vi "AO_6738_Load_Wfm.vi"(8 "error in (no error)":errorcluster, 9 "SOFTWARE Inputs":T2={"Application Directory"=path "D:/S.O.F.T.S/LABVIEW/PIL", "Software Version"="1.0.0", "Data Path"=path "D:/PIRENEA/DATA", "XML Path"=path "D:/PIRENEA/DATA", "XML File Filter"="*.xml", "XML Saved Path"=path "D:/PIRENEA/DATA/SAVED", "Excit Scripts Path"=path "D:/PIRENEA/TECHNICAL/EXCIT_SCRIPTS", "Excit Scripts File Filter"="*.txt", "Excit Waveforms Path"=path "D:/PIRENEA/TECHNICAL/EXCIT_WFMS", "Excit Waveforms File Filter"="*.bin", "Timing Scripts Path"=path "D:/PIRENEA/TECHNICAL/TIMING_SCRIPTS", "Timing Scripts File Filter"="*.txt", "Timing Waveforms Path"=path "D:/PIRENEA/TECHNICAL/TIMING_WFMS", "Timing Waveforms File Filter"="*.bin", "Trapping Waveforms Path"=path "D:/PIRENEA/TECHNICAL/TRAPPING_WFMS", "Trapping Waveforms File Filter"="*.bin"}, 10 "RF_TRAPPING Inputs":T1={"Init Values"=[0.0, 1.0, 1.0, 0.0], "Opening Values"=[0.0, -4.0, 1.0, 0.0], "Trapping Values"=[0.0, 1.0, 1.0, 0.0], "Emptying Values"=[0.0, 1.0, -7.0, 0.0], "RF Trap ON"=FALSE, "RF Accums"=1, "Number of Voltages"=4} {"RF Accums" min=1 max=100; "Trapping Values" min=-10.0 max=10.0; "Init Values" min=-10.0 max=10.0; "Emptying Values" min=-10.0 max=10.0; "Opening Values" min=-10.0 max=10.0}, 11 "Instrument handle in":refnum<k21> caption="tâche/voies en entrée") -> (0 "error out":errorcluster, 1 "number of samples written per channel":u32 caption="nombre d'échantillons écrits par voie", 2 "number of samples":i32, 3 "Instrument handle out":refnum<k21>)   [LabVIEW 2024]
doc: "This VI demonstrates how to load dynamic waveforms into the board.\n\n1. The waveform binary files are read one by one from the waveform folder.\n2. The data are converted to U32 format and loaded into the on-board memory.\n\nThis VI returns the max memory size of the board, the memory used after loading, and a list of the waveforms loaded. No check of memory overflow is done."
uses:
  controls/SOFTWARE_Inputs.ctl
  controls/RF_TRAPPING_Inputs.ctl
  <vilib>/DAQmx/write.llb/DAQmx Write (Analog 2D DBL NChan NSamp).vi
  <vilib>/DAQmx/miscellaneous.llb/DAQmx Fill In Error Info.vi
  <resource>/objmgr/daqmx.rc
panel:
  # "RF_V1"
  # "RF_V2"
  # "RF_V3"
  # "RF_V4"
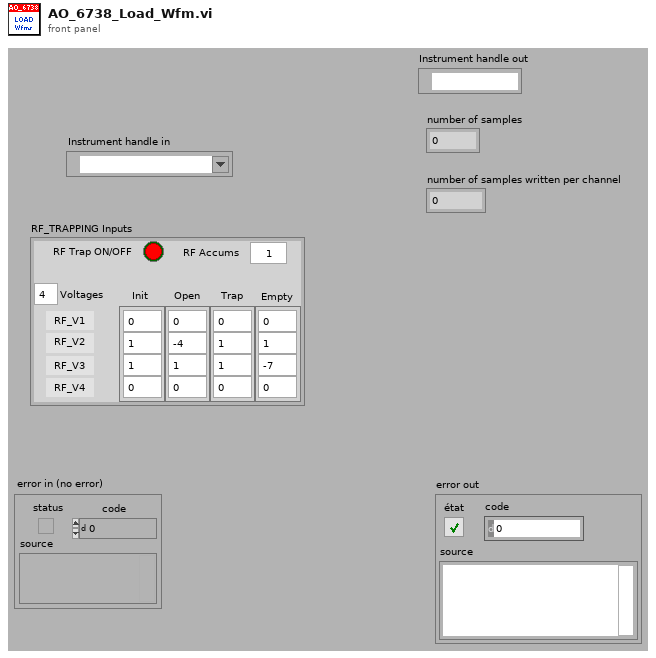
[diagram p1: front panel]
types:
  T1 = typedef "RF_TRAPPING_Inputs.ctl" = cluster{"Init Values":dbl[], "Opening Values":dbl[], "Trapping Values":dbl[], "Emptying Values":dbl[], "RF Trap ON":bool, "RF Accums":i32, "Number of Voltages":i32}
  T2 = typedef "SOFTWARE_Inputs.ctl" = cluster{"Application Directory":path, "Software Version":string, "Data Path":path, "XML Path":path, "XML File Filter":string, "XML Saved Path":path, "Excit Scripts Path":path, "Excit Scripts File Filter":string, "Excit Waveforms Path":path, "Excit Waveforms File Filter":string, "Timing Scripts Path":path, "Timing Scripts File Filter":string, "Timing Waveforms Path":path, "Timing Waveforms File Filter":string, "Trapping Waveforms Path":path, "Trapping Waveforms File Filter":string}
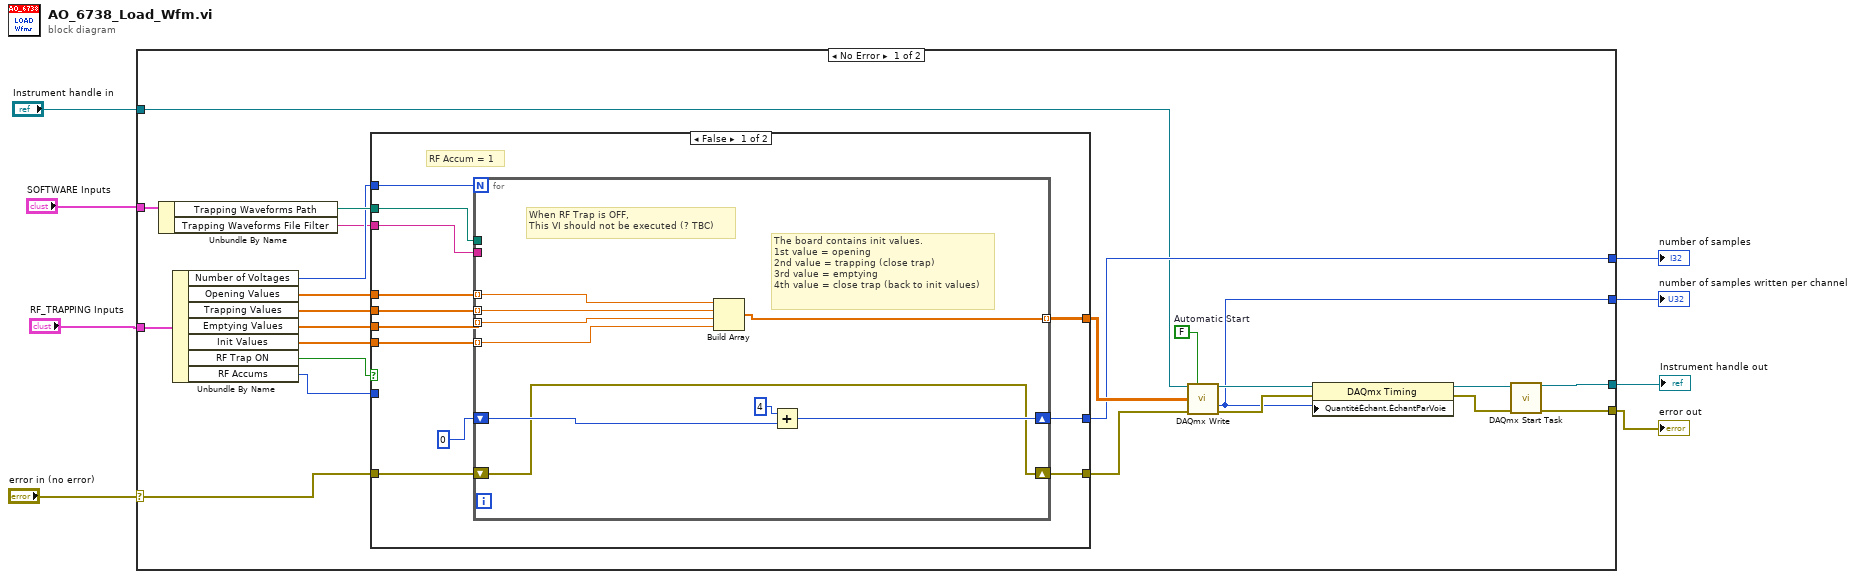
[diagram p0: block diagram]
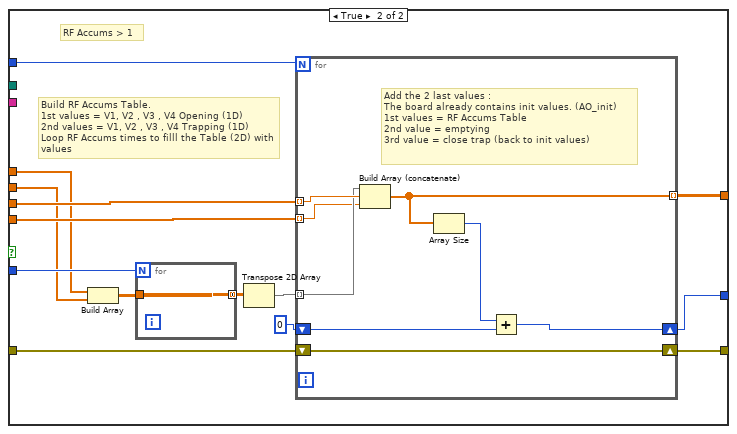
[diagram p2: hidden frame]
diagram:
  n1 = case shown="No Error" "error in (no error)" {
    selector: "error in (no error)" -> [w18 w78]
    tunnel: [w23 w78] -> w8
    tunnel: "SOFTWARE Inputs" -> [w32 _]
    tunnel: [w22 _] -> w7
    tunnel: [w12 _] -> w6
    tunnel: "Instrument handle in" -> [w21 w77]
    tunnel: [w17 w77] -> w3
    tunnel: "RF_TRAPPING Inputs" -> [w9 _]
    frame No Error {
      w31 = FALSE  # Automatic Start
      n2 = Unbundle By Name(w32) -> ("Trapping Waveforms Path"=w29:path, "Trapping Waveforms File Filter"=w20:string)
      n3 = Unbundle By Name(w9) -> ("Number of Voltages"=w28:i32, "Opening Values"=w26:dbl[], "Trapping Values"=w25:dbl[], "Emptying Values"=w27:dbl[], "Init Values"=w24:dbl[], "RF Trap ON"=w11:bool, "RF Accums"=w10:i32)
      n4 = case shown="False" w11 {
        tunnel: [w44 w57] -> w30
        tunnel: w29 -> [w42 _]
        tunnel: w28 -> [w33 w54]
        tunnel: w27 -> [w41 w64]
        tunnel: w26 -> [w40 w56]
        tunnel: w25 -> [w39 w55]
        tunnel: w24 -> [w38 w63]
        tunnel: [w37 w58] -> w22
        tunnel: w20 -> [w36 _]
        tunnel: [w35 w60] -> w19
        tunnel: w18 -> [w34 w61]
        tunnel: w10 -> [_ w65]
        frame False {
          # "RF Accum = 1"
          n5 = for {
            N: w33 -> [_]
            tunnel: w40 -> [w52] mode=indexing
            tunnel: w41 -> [w51] mode=indexing
            tunnel: w39 -> [w50] mode=indexing
            tunnel: [w53] -> w44 mode=indexing
            tunnel: w42 -> [_]
            shift-right: [w48] -> w37
            shift-left: 0 -> [w49]
            tunnel: w38 -> [w47] mode=indexing
            tunnel: w36 -> [_]
            shift-right: [w46] -> w35
            shift-left: w34 -> [w46]
            # "When RF Trap is OFF,\nThis VI should not be executed (? TBC)"
            # "The board contains init values.\n1st value = opening\n2nd value = trapping (close trap)\n3rd value = emptying\n4th value = close trap (back to init values)"
            n6 = Build Array(w52, w50, w51, w47) -> (w53:dbl[])
            n7 = Add(x=4, y=w49) -> (x+y=w48:i32)
          }
        }
        frame True {
          # "Build RF Accums Table.\n1st values = V1, V2 , V3 , V4 Opening (1D)\n2nd values = V1, V2 , V3 , V4 Trapping (1D)\nLoop RF Accums times to filll the Table (2D) with  values"
          # "RF Accums > 1"
          n8 = Build Array(w56, w55) -> (w67:dbl[][])
          n9 = for {
            N: w65 -> [_]
            tunnel: w67 -> [w76]
            tunnel: [w76] -> w66 mode=concatenating
          }
          n10 = Transpose 2D Array(2D array=w66) -> (transposed array=w62:dbl[][])
          n11 = for {
            N: w54 -> [_]
            tunnel: w64 -> [w75] mode=indexing
            tunnel: w62 -> [w74] mode=indexing
            tunnel: [w69] -> w57 mode=indexing
            shift-right: [w72] -> w58
            shift-left: 0 -> [w73]
            tunnel: w63 -> [w71] mode=indexing
            shift-right: [w70] -> w60
            shift-left: w61 -> [w70]
            # "Add the 2 last values :\nThe board already contains init values. (AO_init)\n1st values = RF Accums Table\n2nd value = emptying\n3rd value = close trap (back to init values)"
            n12 = Build Array (concatenate)(w74, w75, w71) -> (w69:dbl[])
            n13 = Array Size(array=w69) -> (size(s)=w68:i32)
            n14 = Add(x=w68, y=w73) -> (x+y=w72:i32)
          }
        }
      }
      n15 = call-poly <vilib>:"DAQmx Write.vi"("task/channels in"=w21, "auto start"=w31, "data"=w30, "error in"=w19) -> ("task out"=w16:refnum<k21>, "number of samples written per channel"=w12:u32, "error out"=w14:errorcluster)  [unwired: 9 in]
      n16 = property class="DAQmx Timing"(reference=w16, error in=w14, "QuantitéÉchant.ÉchantParVoie"=w12) -> (reference out=w15:refnum<k21>, error out=w13:errorcluster)
      n17 = call <vilib>:"DAQmx Start Task.vi"("task/channels in"=w15, "error in"=w13) -> ("task out"=w17:refnum<k21>, "error out"=w23:errorcluster)  [unwired: 12 in]
    }
    frame Error {
    }
  }
  "error out" <- w8
  "number of samples" <- w7
  "number of samples written per channel" <- w6
  "Instrument handle out" <- w3
